vi "Encoder.vi"(11 "Reset Encoder?":bool) -> (0 "Encoder Rate (deg/sec)":dbl, 1 "Encoder Direction":string, 2 "revolutions":dbl, 3 "Current angle (deg)":dbl(knob) scale=0.0..360.0)   [LabVIEW 2015]
panel:
  out "Encoder Alarm Status":string
  out "Distance (in)":dbl
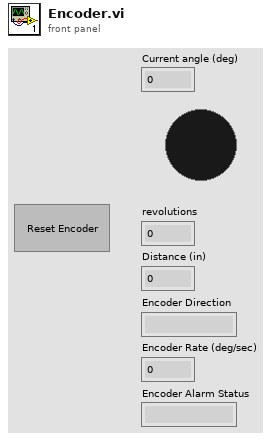
[diagram p1: front panel]
types:
  T1 = typedef "WPI_EncoderDevRef.ctl" = cluster{"DevStatus":errorcluster, "EncoderIndex":T2, "CounterIndex":T3, "DistancePerCount":dbl, "Decoding Type":T4}
  T2 = typedef "FPGA_EncoderIdx.ctl" = enum8{"Enc 0", "Enc 1", "Enc 2", "Enc 3", "Enc 4", "Enc 5", "Enc 6", "Enc 7", "Invalid"}
  T3 = typedef "FPGA_CounterCtrSystemIndex.ctl" = enum8{"Ctr 0", "Ctr 1", "Ctr 2", "Ctr 3", "Ctr 4", "Ctr 5", "Ctr 6", "Ctr 7", "Invalid"}
  T4 = typedef "WPI_EncoderType.ctl" = enum16{"1x", "2x", "4x"}
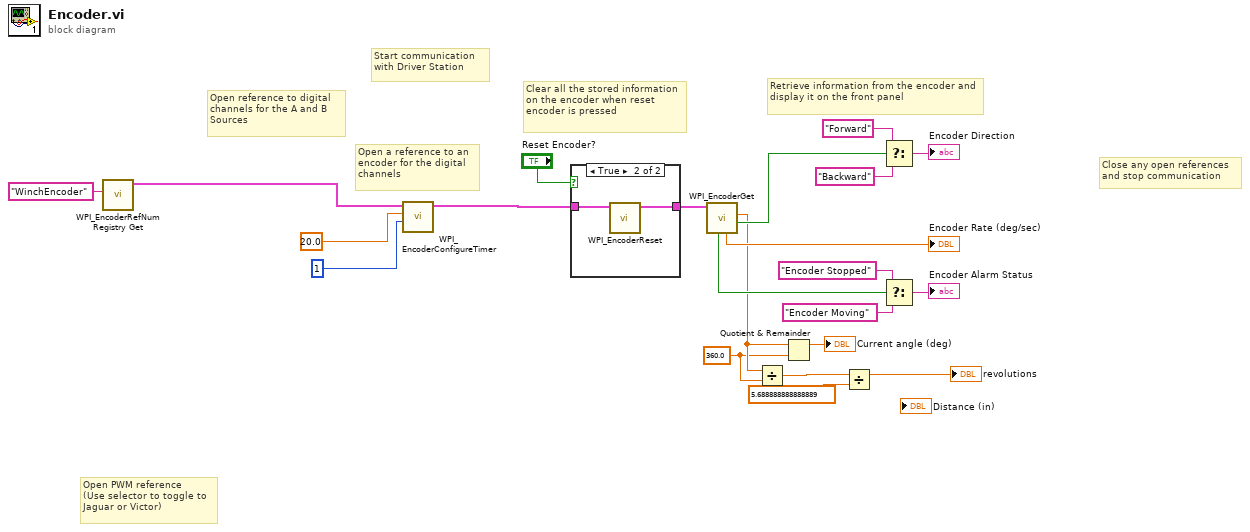
[diagram p0: block diagram]
diagram:
  w8 = 360.0 ("y")
  # "Retrieve information from the encoder and display it on the front panel"
  # "Clear all the stored information on the encoder when reset encoder is pressed"
  # "Open PWM reference\n(Use selector to toggle to Jaguar or Victor)"
  # "Start communication with Driver Station"
  # "Close any open references\nand stop communication"
  # "Open a reference to an\nencoder for the digital \nchannels"
  # "Open reference to digital \nchannels for the A and B\nSources"
  n1 = call <vilib>:"WPI_EncoderRefNum Registry Get.vi"("refnum name"="WinchEncoder") -> ("EncoderDevRef"=w3:T1)  [unwired: 9 in, 1 out]
  n2 = call <vilib>:"WPI_EncoderConfigureTimer.vi"("Number Samples to Average"=u8 1, "Minimum Rate"=20.0, "EncoderDevRef"=w3) -> ("EncoderDevRef"=w22:T1)  [unwired: 1 in, 7 out]
  n3 = case shown="True" "Reset Encoder?" {
    tunnel: w22 -> [w23 w25]
    tunnel: [w23 w24] -> w18
    frame False {
    }
    frame True {
      n4 = call <vilib>:"WPI_EncoderReset.vi"("EncoderDevRef"=w25) -> ("EncoderDevRef"=w24:T1)  [unwired: 1 in, 9 out]
    }
  }
  n5 = call <vilib>:"WPI_EncoderGet.vi"("EncoderDevRef"=w18) -> ("Direction"=w17:bool, "Distance"=w9:dbl, "Rate"=→"Encoder Rate (deg/sec)":dbl, "Stopped"=w16:bool)  [unwired: 1 in, 6 out]
  n6 = Divide(x=w9, y=w8) -> (x/y=w7:dbl)
  n7 = Quotient & Remainder(x=w9, y=w8) -> (x-y*floor(x/y)=→"Current angle (deg)":dbl)  [unwired: 1 out]
  n8 = Divide(x=w7, y=5.688888888888889) -> (x/y=→"revolutions":dbl)
  n9 = Select(t="Forward", s=w17, f="Backward") -> (s? t:f=→"Encoder Direction":string)
  n10 = Select(t="Encoder Stopped", s=w16, f="Encoder Moving") -> (s? t:f=→"Encoder Alarm Status":string)
